vi "LJM logger add data to file.vi"(10 "Data":string, 11 "file path":path) -> (0 "error":bool)   [LabVIEW 2026]
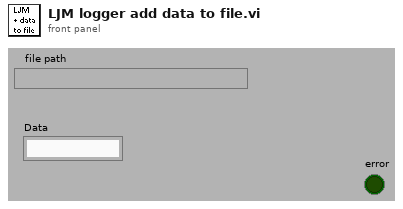
[diagram p1: front panel]
types:
  T1 = enum16{"open", "open or create", "create or replace", "create", "open (read only)"}
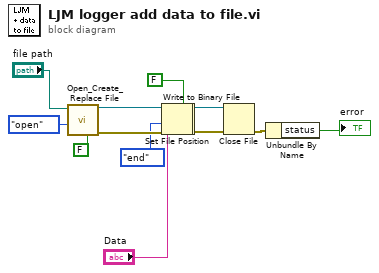
[diagram p0: block diagram]
diagram:
  n1 = call <vilib>:"Open_Create_Replace File.vi"("advisory dialog? (display:T)"=FALSE, "function (open:0)"=T1."open", "file path"="file path") -> ("error out"=w11:errorcluster, "refnum"=w12:refnum<file>)  [unwired: 5 in, 2 out]
  n2 = Set File Position(refnum=w12, from (0:start)=enum16{"start", "end", "current"}."end" ("pos mode (0:2)"), error in=w11) -> (refnum out=w3:refnum<file>, error out=w2:errorcluster)  [unwired: 1 in]
  n3 = Write to Binary File(file (use dialog)=w3, data="Data", error in=w2, 5:FALSE ("prepend array or string size? (T)")) -> (refnum out=w14:refnum<file>, error out=w13:errorcluster)  [unwired: 2 in, 1 out]
  n4 = Close File(refnum=w14, error in=w13) -> (error out=w6:errorcluster)  [unwired: 1 out]
  n5 = Unbundle By Name(w6) -> ("status"=→"error":bool)
